vi "ReadDebugFifo-1.vi"(8 "error in (no error)":errorcluster, 11 "FpgaInterface in":refnum<class "FpgaInterface.lvclass">) -> (0 "error out":errorcluster, 2 "Data":u32[](array[numeric]), 3 "FpgaInterface out":refnum<class "FpgaInterface.lvclass">)   [LabVIEW 2017, in "FpgaInterface.lvclass"]
uses:
  FpgaInterface.lvclass
  FpgaInterface.lvclass/FpgaInterface.ctl
  <vilib>/Utility/error.llb/Error Cluster From Error Code.vi
  <vilib>/rvi/errors/niLvFpgaAdjustHostInterfaceError.vi
  <vilib>/rvi/interface/nirviMethod/nirviMethod.xnode
  <vilib>/FPGAPlugInAG/Dynamic/niLvFpga_ReadFifo_Dynamic.vi
  <vilib>/rvi/errors/niLvFpgaMergeErrorWithErrorCode.vi
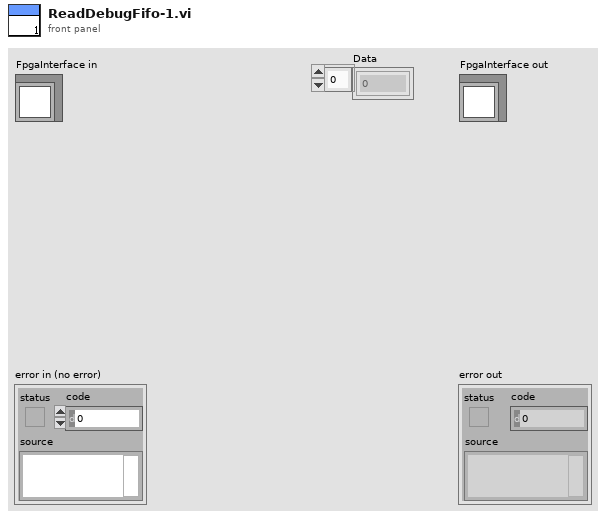
[diagram p1: front panel]
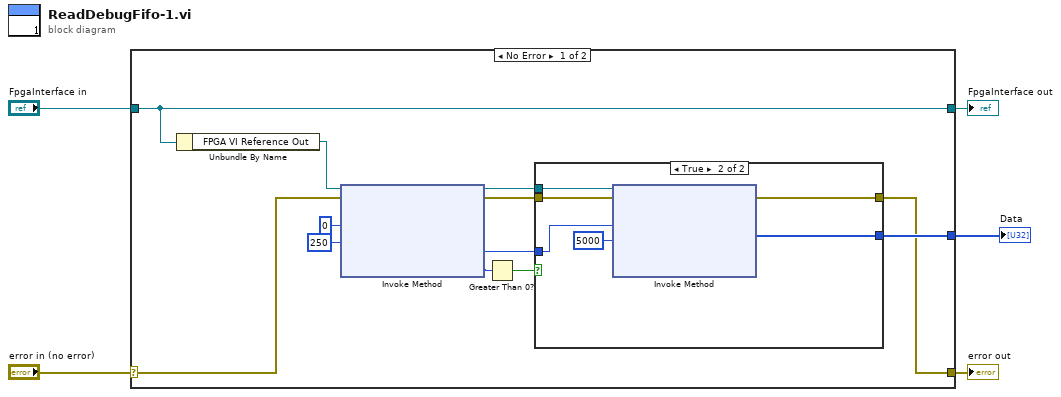
[diagram p0: block diagram]
diagram:
  n1 = case shown="No Error" "error in (no error)" {
    selector: "error in (no error)" -> [w15 w25]
    tunnel: [w7 w25] -> w4
    tunnel: [w16 w24] -> w2
    tunnel: "FpgaInterface in" -> [w16 w24]
    tunnel: [w8 _] -> w1
    frame No Error {
      n2 = Unbundle By Name(w16) -> ("FPGA VI Reference Out"=w6:refnum<k20>)
      n3 = xnode "Invoke Method"("FPGA VI Reference In"=w6, "error in"=w15, "Number of Elements"=u32 0, "Timeout (ms)"=250) -> ("FPGA VI Reference Out"=w10:refnum<k20>, "error out"=w11:errorcluster, "Elements Remaining"=w9:u32)  [unwired: 1 out]
      n4 = Greater Than 0?(x=w9) -> (x > 0?=w12:bool)
      n5 = case shown="True" w12 {
        tunnel: w11 -> [w17 w23]
        tunnel: w10 -> [_ w22]
        tunnel: w9 -> [_ w21]
        tunnel: [_ w19] -> w8
        tunnel: [w17 w18] -> w7
        frame False {
        }
        frame True {
          n6 = xnode "Invoke Method"("FPGA VI Reference In"=w22, "error in"=w23, "Number of Elements"=w21, "Timeout (ms)"=5000) -> ("error out"=w18:errorcluster, "Data"=w19:u32[])  [unwired: 2 out]
        }
      }
    }
    frame Error {
    }
  }
  "error out" <- w4
  "FpgaInterface out" <- w2
  "Data" <- w1
